vi "LastElementDbl.vi"(1 "array":dbl[](array[numeric]) format="%.2f") -> (0 "Numeric":dbl format="%.2f")   [LabVIEW 2009]
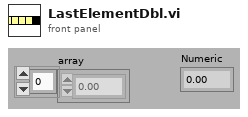
[diagram p1: front panel]
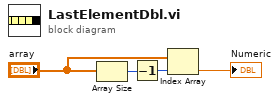
[diagram p0: block diagram]
diagram:
  n1 = Array Size(array="array") -> (size(s)=w1:i32)
  n2 = Decrement(x=w1) -> (x-1=w2:i32)
  n3 = Index Array(array="array", index=w2) -> (element=→"Numeric":dbl)
